vi "Update Progress Bar Value.vi"(9 "Data in":T1 caption="Data In", 10 "Container State":T2, 11 "Display State in":T3={"Window Handle"=refnum, "Maximum"=0, "State Change Action"=enum."Method - Initialize", "Running"=FALSE, "Visable Items"={"Label"=TRUE, "Caption"=FALSE}, "Value"=100, "Show Progress Bar"=FALSE} caption="State") -> (0 "Coerced?":bool, 1 "Data Out":T1, 3 "Display State out":T3={"Window Handle"=refnum, "Maximum"=0, "State Change Action"=enum."Method - Initialize", "Running"=FALSE, "Visable Items"={"Label"=TRUE, "Caption"=FALSE}, "Value"=100, "Show Progress Bar"=FALSE} caption="State")   [LabVIEW 2011, in "Taskbar Progress Bar.xctl"]
uses:
  Taskbar Progress Bar.xctl
  Abilities/PB State.ctl
  TypeDefs/Dispaly State Change Methods.ctl
  Abilities/PB Data.ctl
  <vilib>/_xctls/Container State.ctl
  <vilib>/TaskbarProgressAPI/_TypeDefs/Progress State.ctl
  <vilib>/TaskbarProgressAPI/TaskbarProgressAPI.lvlib
  <vilib>/_xctls/XControlSupport.lvlib
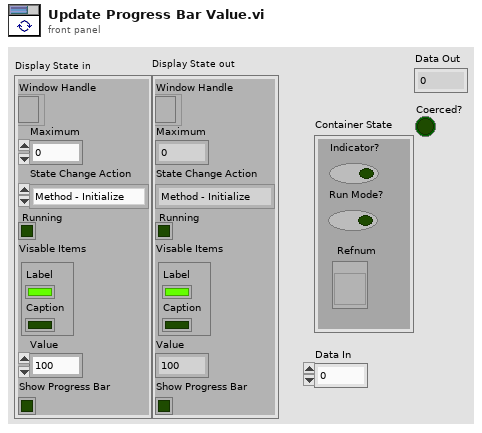
[diagram p1: front panel]
types:
  T1 = typedef "Taskbar Progress Bar.xctl/PB Data.ctl" = u64
  T2 = typedef "XControlSupport.lvlib/Container State.ctl" = cluster{"Indicator?":bool, "Run Mode?":bool, " Refnum":refnum<vi>}
  T3 = typedef "Taskbar Progress Bar.xctl/PB State.ctl" = cluster{"Window Handle":refnum<k24>, "Maximum":u64, "State Change Action":T4, "Running":bool, "Visable Items":cluster{"Label":bool, "Caption":bool}, "Value":u64, "Show Progress Bar":bool}
  T4 = typedef "Taskbar Progress Bar.xctl/Dispaly State Change Methods.ctl" = enum16{"No Action", "Created", "Method - Initialize", "Method - Increment", "Method - Pause", "Method - Error", "Method - Finish", "Property - Show Progress Bar"}
  T5 = typedef "TaskbarProgressAPI.lvlib/Progress State.ctl" = i32
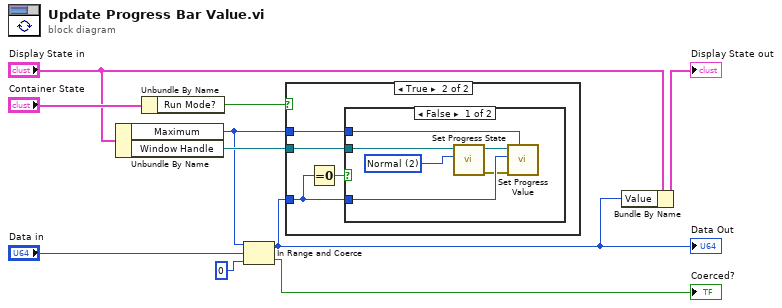
[diagram p0: block diagram]
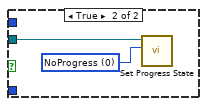
[diagram p3: hidden frame]
diagram:
  n1 = Unbundle By Name("Display State in") -> ("Maximum"=w5:u64, "Window Handle"=w6:refnum<k24>)
  n2 = Unbundle By Name("Container State") -> ("Run Mode?"=w10:bool)
  n3 = In Range and Coerce(upper limit=w5, x="Data in", lower limit=T1 0) -> (coerced(x)=w1:T1, In Range?=→"Coerced?":bool)
  "Data Out" <- w1
  n4 = case shown="True" w10 {
    tunnel: w6 -> [_ w13]
    tunnel: w1 -> [_ w12]
    tunnel: w5 -> [_ w14]
    frame False {
    }
    frame True {
      n5 = Equal To 0?(x=w12) -> (x = 0?=w11:bool)
      n6 = case shown="False" w11 {
        tunnel: w14 -> [w20 _]
        tunnel: w13 -> [w19 w22]
        tunnel: w12 -> [w17 _]
        frame False {
          w16 = T5 2 items=["NoProgress"=0, "Indeterminate"=1, "Normal"=2, "Error"=4, "Paused"=8] ("State (No Progress)")
          n7 = call <vilib>:"Set Progress State.vi"("State (No Progress)"=w16, "Window Handle"=w19) -> ("error out"=w15:errorcluster, "dup Window Handle"=w18:refnum<k24>)  [unwired: 8 in]
          n8 = call <vilib>:"Set Progress Value.vi"("maximum (100)"=w20, "error in (no error)"=w15, "current (0)"=w17, "Window Handle"=w18) -> ()  [unwired: 6 in, 2 out]
        }
        frame True {
          w21 = T5 0 items=["NoProgress"=0, "Indeterminate"=1, "Normal"=2, "Error"=4, "Paused"=8] ("State (No Progress)")
          n9 = call <vilib>:"Set Progress State.vi"("State (No Progress)"=w21, "Window Handle"=w22) -> ()  [unwired: 8 in, 2 out]
        }
      }
    }
  }
  n10 = Bundle By Name(cluster="Display State in", "Value"=w1) -> (→"Display State out":T3)
